vi "USRP_RA_molecularLine_monitor_multSamples.vi"() -> ()   [LabVIEW 2016]
doc: "USRP maser line receiver for amateur radio astronomy."
uses:
  <vilib>/Analysis/4window.llb/windowTd.ctl
  <vilib>/Utility/error.llb/DialogType.ctl
  <vilib>/Analysis/3filter.llb/Filter Passband Type.ctl
  <vilib>/Analysis/2dsp.llb/Power Spectrum (CDB).vi
  <vilib>/Analysis/5stat.llb/RMS (CDB).vi
  <vilib>/Utility/config.llb/Read Key (Double).vi
  <instrlib>/niUSRP/niUSRP Fetch Rx Data (I16).vi
  <vilib>/Analysis/3filter.llb/Butterworth Filter (CDB).vi
  <vilib>/Analysis/0measdsp.llb/Scaled Time Domain Window (CDB).vi
  <vilib>/Utility/file.llb/Write Delimited Spreadsheet (DBL).vi
  <vilib>/Utility/config.llb/Write Key (Double).vi
  <vilib>/Analysis/NI_AALBase.lvlib
  <vilib>/Utility/config.llb/NI_LVConfig.lvlib
  <vilib>/Analysis/NI_AALPro.lvlib
panel:
  in  "Set_mult":bool caption="Set mult"
  in  "Tsys":dbl=150.0 caption="Tsys, K" format="%#_13g"
  in  "Reference Frequency Source":string(combo)="Internal" caption="Ref Freq Source"
  in  "FFT_window":T1=2 caption="FFT window" items=["Rectangle"=0, "Hanning"=1, "Hamming"=2, "Blackman-Harris"=3, "Exact Blackman"=4, "Blackman"=5, "Flat Top"=6, "4 Term B-Harris "=7, "7 Term B-Harris"=8, "Low Sidelobe"=9, "Blackman Nuttall"=11, "Triangle"=30, "Bartlett-Hanning"=31, "Bohman"=32, "Parzen"=33, "Welch"=34, "Kaiser"=60, "Dolph-Chebyshev"=61, "Gaussian"=62]
  out "coerced gain, dB":dbl format="%#_6f"
  in  "Bandwidth_MHz":dbl=2.0 caption="Bandwidth, MHz" min=0.1 max=64.0
  in  "Frequency_MHz":dbl(knob)=1427.4 caption="Frequency, MHz" min=70.0 max=6000.0 scale=70.0..6000.0 scale format="%#1_5g"
  out "Active Antenna":string
  out "Freq (actual)":dbl=1431299999.9970195 format="%#.6p"
  in  "device ID":refnum<k15>="B200miniUSRP"
  out "FFT_error":i32 caption="FFT, proc"
  in  "FFT_size_mult":dbl=50000.0 caption="FFT size av multiplier" min=1.0 max=100000.0 step=1.0 format="%#_8g"
  in  "Power mult":dbl=7e-06 format="%#_13g"
  out "Power_diff":dbl caption="Power diff"
  out "Power_ref":dbl caption="Power ref"
  in  "Power ref":bool
  out "Power_BW":dbl caption="Power in BW"
  out "RMS_error":i32 caption="RMS"
  in  "Pause":bool
  in  "cycle delay, ms":u32
  in  "dB_scale":bool caption="dB scale"
  in  "Reset":bool
  out "TIme elapsed, s":dbl
  in  "Rewrite":bool
  out "Number of av":u32
  in  "File recording":bool
  out "cycle time, s":dbl
  out "Overload":bool
  out "Level":dbl(slide) scale=0.0..1.0 scale format="%#_3g"
  in  "Video_av_on":bool
  in  "Video_av":dbl=500.0 caption="Video Av" min=1.0 max=1000000.0 step=1.0 format="%#_4g"
  in  "DC_block":bool caption="DC block"
  in  "Freq_cutoff_kHz":dbl=10.0 caption="Cutoff, kHz" min=0.01 max=5000.0 step=1.0
  out "RBW":dbl=4.0 caption="RBW, kHz"
  in  "Plot_mult":dbl=0.00020000000000042206 caption="Plot mult" min=0.0 step=5.0
  in  "?":bool
  out "Samplerate":dbl=20000000.0 caption="Sample rate (SR)" min=80000.0 max=40000000.0 step=1.0 format="%#_8g"
  in  "FFT_size":dbl=501.0 caption="FFT size" min=128.0 max=28000000.0 step=1.0 format="%#_8g"
  in  "VGA1_dB":dbl=19.0 caption="Gain, dB" min=-50.0 max=100.0 step=1.0 format="%#_2g"
  out "Spectrum":cluster{dbl, dbl, dbl[]}(graph)={434.616665995587, 1.9999999937668345e-05, array[5000 elements]} caption="Power Spectrum"
  # "errors (0 if OK)"
  # "noise equivalent"
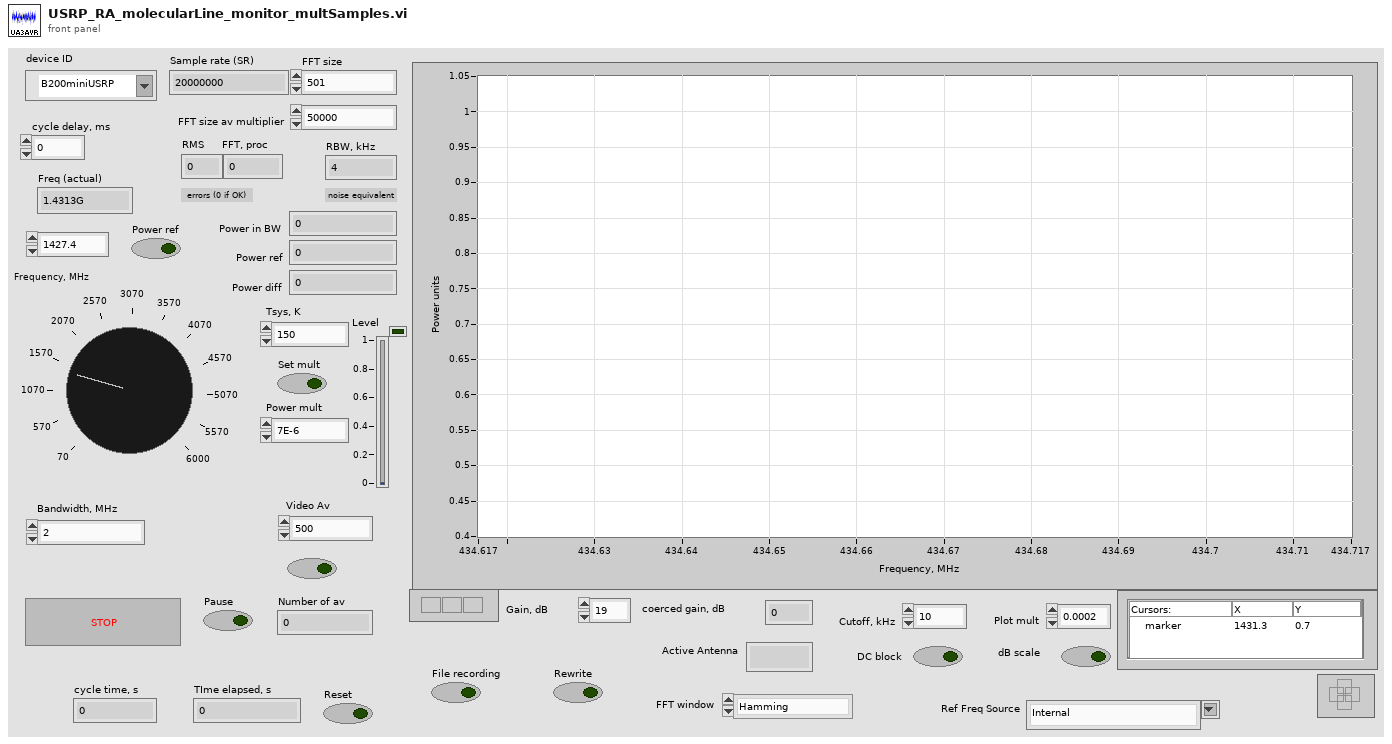
[diagram p1: front panel]
types:
  T1 = typedef "NI_AALPro.lvlib/windowTd.ctl" = u32
  T2 = typedef "DialogType.ctl" = u16
  T3 = typedef "NI_LVConfig.lvlib/Config Data RefNum.ctl" = refnum<k1>
  T4 = typedef "NI_AALBase.lvlib/Filter Passband Type.ctl" = enum32{"Lowpass", "Highpass", "Bandpass", "Bandstop"}
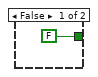
[diagram p3: hidden frame]
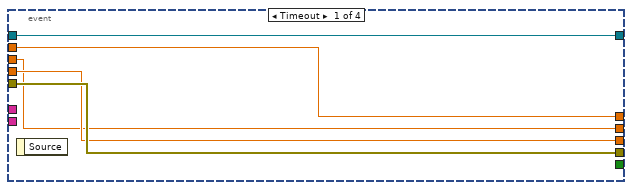
[diagram p4: hidden frame]
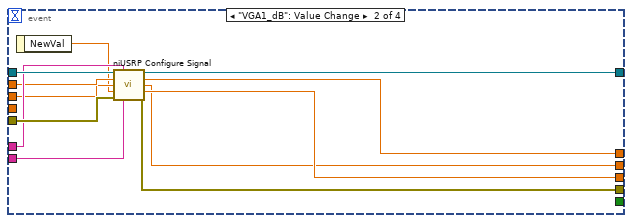
[diagram p5: hidden frame]
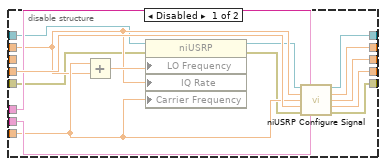
[diagram p6: hidden frame]
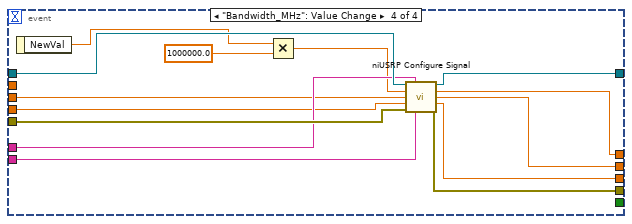
[diagram p7: hidden frame]
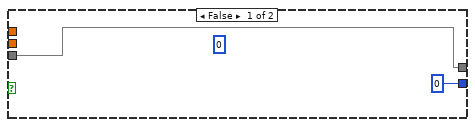
[diagram p8: hidden frame]
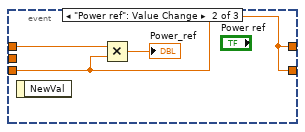
[diagram p9: hidden frame]
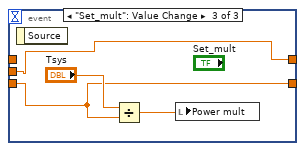
[diagram p10: hidden frame]
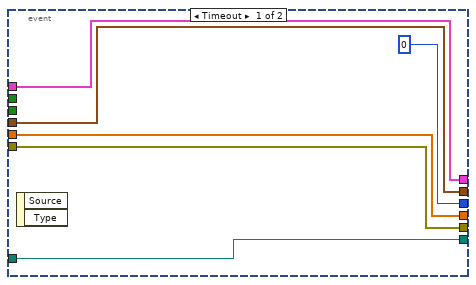
[diagram p11: hidden frame]
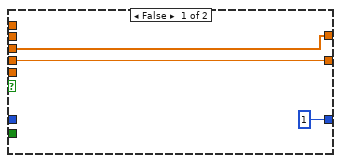
[diagram p13: hidden frame]
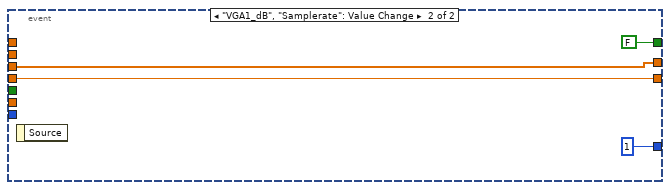
[diagram p15: hidden frame]
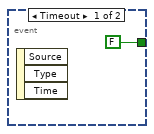
[diagram p16: hidden frame]
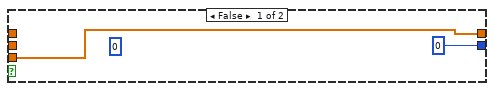
[diagram p17: hidden frame]
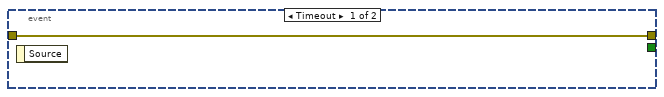
[diagram p18: hidden frame]
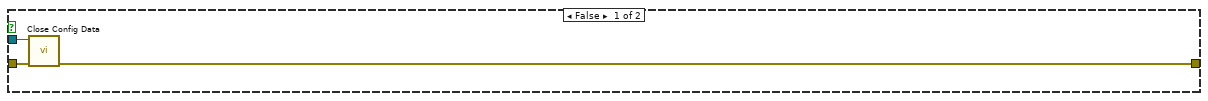
[diagram p20: hidden frame]
diagram:
  w24 = 16 items=["16-bit"=16, "8-bit"=8] ("Sample Width")
  w25 = 1 items=["CDB", "I16"] ("Host Data Type")
  w11 = "0"  # enabled channel
  w45 = T2 3 items=["no dialog", "OK message", "continue or stop message", "OK message + warnings", "continue/stop + warnings"] ("type of dialog (OK msg:1)")
  w53 = TRUE ("use system decimal point (T)")
  w52 = "Data" ("section")
  # "USRP initialization"
  # "Loag CFG values"
  # "Saving file on Stop"
  # "Reading and loading previously saved parameters from CFG-file"
  # "Saving last parameters to CFG-file"
  n1 = call <vilib>:"Application Directory.vi"() -> ("Application Directory"=w78:path)
  n2 = Build Path(base path=w78, name or relative path="USRP_line_monitor.cfg") -> (appended path=w87:path)
  n3 = call <vilib>:"Open Config Data.vi"("create file if necessary (T)"=TRUE, "configuration file path"=w87) -> ("error out"=w84:errorcluster, "file created?"=w82:bool, "refnum"=w86:T3)  [unwired: 7 in]
  n4 = Not(x=w82) -> (.not. x?=w81:bool)
  n5 = case shown="True" w81 {
    tunnel: w86 -> [w95 w131]
    tunnel: w84 -> [w97 w130]
    tunnel: [w96 w129] -> w44
    frame False {
      n6 = call <vilib>:"Close Config Data.vi"("error in (no error)"=w97, "refnum"=w95) -> ("error out"=w96:errorcluster)  [unwired: 8 in, 1 out]
    }
    frame True {
      w108 = "Data" ("section")
      n7 = call-poly <vilib>:"Read Key.vi"("section"=w108, "error in (no error)"=w130, "key"="Frequency_MHz", "refnum"=w131) -> ("error out"=w104:errorcluster, "value"=w102:dbl, "refnum out"=w105:T3)  [unwired: 4 in, 1 out]
      n8 = property on="Frequency_MHz" class="Knob (strict)"(error in=w104, "Value"=w102) -> (error out=w103:errorcluster)  [unwired: 1 in, 1 out]
      n9 = call-poly <vilib>:"Read Key.vi"("section"=w108, "error in (no error)"=w103, "key"="VGA1_dB" ("Control Name"), "refnum"=w105) -> ("error out"=w127:errorcluster, "value"=w128:dbl, "refnum out"=w121:T3)  [unwired: 4 in, 1 out]
      n10 = property on="VGA1_dB" class="DigNum (strict)"(error in=w127, "Value"=w128) -> (error out=w123:errorcluster)  [unwired: 1 in, 1 out]
      n11 = call-poly <vilib>:"Read Key.vi"("section"=w108, "error in (no error)"=w123, "key"="FFT_size" ("Control Name"), "refnum"=w121) -> ("error out"=w125:errorcluster, "value"=w124:dbl, "refnum out"=w119:T3)  [unwired: 4 in, 1 out]
      n12 = property on="FFT_size" class="DigNum (strict)"(error in=w125, "Value"=w124) -> (error out=w120:errorcluster)  [unwired: 1 in, 1 out]
      n13 = call-poly <vilib>:"Read Key.vi"("section"=w108, "error in (no error)"=w120, "key"="Bandwidth_MHz" ("Control Name"), "refnum"=w119) -> ("error out"=w101:errorcluster, "value"=w99:dbl, "refnum out"=w115:T3)  [unwired: 4 in, 1 out]
      n14 = property on="Bandwidth_MHz" class="DigNum (strict)"(error in=w101, "Value"=w99) -> (error out=w100:errorcluster)  [unwired: 1 in, 1 out]
      n15 = call-poly <vilib>:"Read Key.vi"("section"=w108, "error in (no error)"=w100, "key"="Plot_mult" ("Control Name"), "refnum"=w115) -> ("error out"=w117:errorcluster, "value"=w116:dbl, "refnum out"=w109:T3)  [unwired: 4 in, 1 out]
      n16 = property on="Plot_mult" class="DigNum (strict)"(error in=w117, "Value"=w116) -> (error out=w110:errorcluster)  [unwired: 1 in, 1 out]
      n17 = call-poly <vilib>:"Read Key.vi"("section"=w108, "error in (no error)"=w110, "key"="Video_av" ("Control Name"), "refnum"=w109) -> ("error out"=w112:errorcluster, "value"=w111:dbl, "refnum out"=w107:T3)  [unwired: 4 in, 1 out]
      n18 = property on="Video_av" class="DigNum (strict)"(error in=w112, "Value"=w111) -> (error out=w106:errorcluster)  [unwired: 1 in, 1 out]
      n19 = call <vilib>:"Close Config Data.vi"("error in (no error)"=w106, "refnum"=w107) -> ("error out"=w129:errorcluster)  [unwired: 8 in, 1 out]
    }
  }
  n20 = flat-sequence {
    tunnel: w44 -> [w135]
    tunnel: [w135] -> w9
    tunnel: ["VGA1_dB"] -> w8
    tunnel: ["Frequency_MHz"] -> w7
    tunnel: ["Bandwidth_MHz"] -> w6
    frame #0 {
    }
  }
  n21 = Multiply(x=w6, y=1000000.0) -> (x*y=w14:dbl)
  n22 = Multiply(x=w7, y=1000000.0) -> (x*y=w18:dbl)
  n23 = Round To Nearest(number=w14) -> (nearest integer value=w15:dbl)
  n24 = disable-structure shown="Disabled" {
    disable-tunnel: [w138 w139] -> w27
    disable-tunnel: w18 -> [w137 w139]
    disable-tunnel: w15 -> [w136 _]
    frame Disabled {
      n25 = Add(x=w137, y=w136) -> (x+y=w138:dbl)
    }
    frame Enabled {
    }
  }
  n26 = call <instrlib>:"niUSRP Open Rx Session.vi"("device names"="device ID", "reset"=TRUE, "error in (no error)"=w9) -> ("session handle out"=w20:refnum<k15>, "error out"=w30:errorcluster)  [unwired: 11 in]
  n27 = property class="niUSRP"(reference=w20, error in=w30, "Enabled Channels"=w11, "Host Data Type"=w25, "Sample Width"=w24, "Expected Peak"=1.52587890625e-05, "Bandwidth"=60000000.0 ("Configuration:Bandwidth"), "Reference Frequency Source"="Reference Frequency Source", "Timebase Clock Source"="Internal", "Number of Samples Is Finite"=FALSE ("Configuration:Number of Samples Is Finite"), "LO Frequency"=w27, "IQ Rate"=w15, "Carrier Frequency"=w18, "Gain"=w8) -> (reference out=w21:refnum<k15>, error out=w22:errorcluster, "Active Antenna"=w4:string)
  "Active Antenna" <- w4
  n28 = call <vilib>:"Application Directory.vi"() -> ("Application Directory"=w35:path)
  n29 = call <instrlib>:"niUSRP Configure Signal.vi"("session handle"=w21, "channel list"=w11, "IQ rate"=w15, "carrier frequency"=w18, "gain"=w8, "error in (no error)"=w22, "active antenna"=w4) -> ("session handle out"=w12:refnum<k15>, "coerced IQ rate"=w13:dbl, "coerced carrier frequency"=w17:dbl, "coerced gain"=w5:dbl, "error out"=w10:errorcluster)  [unwired: 4 in]
  "Freq (actual)" <- w17
  "coerced gain, dB" <- w5
  n30 = Build Path(base path=w35, name or relative path="samples-data.txt") -> (appended path=w34:path)
  n31 = Get Date/Time In Seconds() -> (seconds since 1Jan1904=w33:timestamp)
  n32 = while {
    tunnel: [w216] -> w2
    shift-right: [w215] -> w74
    shift-left: _ -> [w255]
    tunnel: w34 -> [w220]
    tunnel: w10 -> [w161]
    tunnel: ["File recording"] -> w76
    tunnel: [w217] -> w75
    tunnel: [w214] -> _
    shift-right: [w218] -> _
    shift-left: w33 -> [w225]
    tunnel: [w208] -> w51
    shift-right: [w199] -> _
    shift-left: _ -> [w203]
    shift-right: [w195] -> _
    shift-left: _ -> [w194]
    tunnel: w17 -> [w150]
    tunnel: w13 -> [w153]
    tunnel: w12 -> [w159]
    tunnel: [w174] -> w1
    tunnel: w11 -> [w156]
    tunnel: w5 -> [w147]
    tunnel: w4 -> [w155]
    stop <- w143 stop-if-true
    # "Spectrum processing and indication"
    # "Power in bandwidth indication"
    # "File savings on pause"
    # "Timing"
    # "Noise RBW"
    # "Sampling procedures"
    # "Changing the main parameters on flight"
    # "Power in the bandwidth and overload indication"
    # "Spectrum averaging procedures"
    # "Finish and close BladeRF"
    # "Video averaging"
    n33 = feedback #1(w153) -> (w152:dbl)
    n34 = feedback #2(w150) -> (w149:dbl)
    n35 = feedback #3(w147) -> (w146:dbl)
    n36 = event shown="[2] \"Frequency_MHz\": Value Change" {
      selector: _ -> [_ _ _ _]
      dyn-events: _ -> [_ _ _ _]
      timeout: 0 -> [_ _ _ _]
      tunnel: w161 -> [w270 w282 w286 w330]
      tunnel: [w270 w281 w296 w329] -> w160
      tunnel: w159 -> [w269 w279 w285 w328]
      tunnel: [w269 w280 w295 w327] -> w158
      tunnel: w156 -> [_ w278 w290 w325]
      tunnel: w152 -> [w267 w277 w287 _]
      tunnel: w149 -> [w266 w276 w284 w324]
      tunnel: [w268 w274 w291 w317] -> w148
      tunnel: w146 -> [w268 _ w294 w323]
      tunnel: [w267 w273 w293 w319] -> w154
      tunnel: [w266 w272 w292 w318] -> w151
      tunnel: w155 -> [_ w271 w289 w326]
      tunnel: [_ _ TRUE _] -> w141
      event Timeout {
        n37 = event-data() -> ()  [unwired: 1 in, 1 out]
      }
      event "VGA1_dB": Value Change {
        n38 = event-data() -> ("NewVal"=w275:dbl)  [unwired: 1 in]
        n39 = call <instrlib>:"niUSRP Configure Signal.vi"("session handle"=w279, "channel list"=w278, "IQ rate"=w277, "carrier frequency"=w276, "gain"=w275, "error in (no error)"=w282, "active antenna"=w271) -> ("session handle out"=w280:refnum<k15>, "coerced IQ rate"=w273:dbl, "coerced carrier frequency"=w272:dbl, "coerced gain"=w274:dbl, "error out"=w281:errorcluster)  [unwired: 4 in]
      }
      event "Frequency_MHz": Value Change {
        n40 = event-data() -> ("NewVal"=w288:dbl)  [unwired: 1 in]
        n41 = disable-structure shown="Enabled" {
          disable-tunnel: [w311 w315] -> w296
          disable-tunnel: [w310 w316] -> w295
          disable-tunnel: w294 -> [w309 w312]
          disable-tunnel: [w308 w314] -> w293
          disable-tunnel: [w307 w313] -> w292
          disable-tunnel: [w306 w312] -> w291
          disable-tunnel: w290 -> [w305 _]
          disable-tunnel: w289 -> [w304 _]
          disable-tunnel: w288 -> [w302 _]
          disable-tunnel: w287 -> [w301 w314]
          disable-tunnel: w286 -> [w300 w315]
          disable-tunnel: w285 -> [w298 w316]
          disable-tunnel: w284 -> [_ w313]
          frame Disabled {
            n42 = Add(x=w302, y=w301) -> (x+y=w303:dbl)
            n43 = property class="niUSRP"(reference=w298, error in=w300, "LO Frequency"=w303, "IQ Rate"=w301, "Carrier Frequency"=w302) -> (reference out=w297:refnum<k15>, error out=w299:errorcluster)
            n44 = call <instrlib>:"niUSRP Configure Signal.vi"("session handle"=w297, "channel list"=w305, "IQ rate"=w301, "carrier frequency"=w302, "gain"=w309, "error in (no error)"=w299, "active antenna"=w304) -> ("session handle out"=w310:refnum<k15>, "coerced IQ rate"=w308:dbl, "coerced carrier frequency"=w307:dbl, "coerced gain"=w306:dbl, "error out"=w311:errorcluster)  [unwired: 4 in]
          }
          frame Enabled {
          }
        }
      }
      event "Bandwidth_MHz": Value Change {
        n45 = event-data() -> ("NewVal"=w322:dbl)  [unwired: 1 in]
        n46 = Multiply(x=w322, y=1000000.0) -> (x*y=w320:dbl)
        n47 = call <instrlib>:"niUSRP Configure Signal.vi"("session handle"=w328, "channel list"=w325, "IQ rate"=w320, "carrier frequency"=w324, "gain"=w323, "error in (no error)"=w330, "active antenna"=w326) -> ("session handle out"=w327:refnum<k15>, "coerced IQ rate"=w319:dbl, "coerced carrier frequency"=w318:dbl, "coerced gain"=w317:dbl, "error out"=w329:errorcluster)  [unwired: 4 in]
      }
    }
    n48 = feedback-in #1(w154) -> ()
    n49 = feedback-in #2(w151) -> ()
    n50 = feedback-in #3(w148) -> ()
    n51 = Round To Nearest(number="FFT_size") -> (nearest integer value=w193:dbl)
    n52 = Divide(x=w152, y=w193) -> (x/y=w260:dbl)
    n53 = Multiply(x="FFT_size_mult", y=w193) -> (x*y=w192:dbl)
    n54 = To Long Integer(number="FFT_size_mult") -> (32bit integer=w191:i32)
    n55 = To Quad Integer(1:w192) -> (0:w168:i64)
    n56 = case shown="True" w141 {
      tunnel: [FALSE ("T button?") w264] -> w140
      frame False {
      }
      frame True {
        n57 = Two Button Dialog(message="The application will be stopped. To change a frequency, please, start it again.") -> (T button?=w264:bool)  [unwired: 2 in]
      }
    }
    n58 = local write "Freq (actual)"(w151) -> ()
    n59 = local write "Samplerate"(w154) -> ()
    n60 = local write "coerced gain, dB"(w148) -> ()
    n61 = call <instrlib>:"niUSRP Configure Number of Samples.vi"("session handle"=w158, "number of samples is finite"=TRUE, "number of samples"=w168, "error in (no error)"=w160) -> ("session handle out"=w165:refnum<k15>, "error out"=w167:errorcluster)  [unwired: 10 in]
    n62 = call <instrlib>:"niUSRP Initiate.vi"("session handle"=w165, "error in (no error)"=w167) -> ("session handle out"=w164:refnum<k15>, "error out"=w166:errorcluster)  [unwired: 12 in]
    n63 = event shown="[1] \"FFT_size\": Value Change" {
      selector: _ -> [_ _]
      dyn-events: _ -> [_ _]
      timeout: 0 -> [_ _]
      tunnel: [FALSE TRUE] -> w178
      event Timeout {
        n64 = event-data() -> ()  [unwired: 1 in, 3 out]
      }
      event "FFT_size": Value Change {
        n65 = event-data() -> ()  [unwired: 1 in, 3 out]
      }
    }
    n66 = call-poly <instrlib>:"niUSRP Fetch Rx Data (poly).vi"("session handle"=w164, "channel list"=w156, "number of samples"=w168, "error in (no error)"=w166) -> ("session handle out"=w176:refnum<k15>, "data"=w173:i16[], "error out"=w177:errorcluster)  [unwired: 8 in, 1 out]
    n67 = To Long Integer(number=w193) -> (32bit integer=w190:i32)
    n68 = Decimate 1D Array(w173) -> (w172:i16[], w171:i16[])
    n69 = call <instrlib>:"niUSRP Abort.vi"("session handle"=w176, "error in (no error)"=w177) -> ("session handle out"=w174:refnum<k15>, "error out"=w175:errorcluster)  [unwired: 12 in]
    n70 = Re/Im To Complex(1:w171, 2:w172) -> (0:w170:cdb[])
    n71 = Initialize Array(0.0 ("element"), w190) -> (w182:dbl[])
    n72 = for {
      N: w191 -> [_]
      tunnel: w170 -> [w352]
      tunnel: w190 -> [w350]
      shift-right: [w331] -> w179
      shift-left: w182 -> [w337]
      tunnel: w152 -> [w348]
      shift-right: [w343] -> w188
      shift-left: _ -> [_]
      shift-right: [w341] -> w187
      shift-left: _ -> [_]
      shift-right: [w342] -> w186
      shift-left: _ -> [_]
      shift-right: [w340] -> w185
      shift-left: _ -> [_]
      tunnel: "DC_block" -> [w339]
      tunnel: "Freq_cutoff_kHz" -> [w338]
      i -> [w336]
      # "Averaging"
      # "Array division"
      # "Windowing and FFT"
      n73 = Multiply(x=w350, y=w336) -> (x*y=w351:i32)
      n74 = To Double Precision Float(number=w336) -> (double precision float=w333:dbl)
      n75 = Multiply(x=w337, y=w333) -> (x*y=w335:dbl[])
      n76 = Array Subset(array=w352, index=w351, length=w350) -> (w349:cdb[])
      n77 = case shown="True" w339 {
        tunnel: w349 -> [w354 w362]
        tunnel: w348 -> [_ w361]
        tunnel: [0 ("error") w360] -> w343
        tunnel: [w354 w359] -> w346
        tunnel: w338 -> [_ w355]
        frame False {
          (unwired) 0 ("error")
        }
        frame True {
          # "DC block"
          n78 = Multiply(x=1000.0, y=w355) -> (x*y=w357:dbl)
          n79 = call-poly <vilib>:"Butterworth Filter.vi"("filter type"=Filter_Passband_Type."Highpass", "low cutoff freq: fl"=w357, "sampling freq: fs"=w361, "X"=w362) -> ("error"=w360:i32, "Filtered X"=w359:cdb[])  [unwired: 4 in]
        }
      }
      n80 = Increment(x=w333) -> (x+1=w332:dbl)
      n81 = call-poly <vilib>:"Scaled Time Domain Window.vi"("window"="FFT_window", "X"=w346) -> ("error"=w341:i32, "window properties"=w340:cluster{"eq noise BW":dbl, "coherent gain":dbl}, "Windowed X"=w345:cdb[])  [unwired: 7 in]
      n82 = call-poly <vilib>:"Power Spectrum.vi"("X"=w345) -> ("Power Spectrum"=w344:dbl[], "error"=w342:i32)
      n83 = Add(x=w335, y=w344) -> (x+y=w334:dbl[])
      n84 = Divide(x=w334, y=w332) -> (x/y=w331:dbl[])
    }
    n85 = case shown="True" "DC_block" {
      tunnel: w170 -> [w456 w464]
      tunnel: w152 -> [_ w463]
      tunnel: [0 ("error") w462] -> w181
      tunnel: [w456 w461] -> w202
      tunnel: "Freq_cutoff_kHz" -> [_ w457]
      frame False {
        (unwired) 0 ("error")
      }
      frame True {
        # "DC block"
        n86 = Multiply(x=1000.0, y=w457) -> (x*y=w459:dbl)
        n87 = call-poly <vilib>:"Butterworth Filter.vi"("filter type"=Filter_Passband_Type."Highpass", "low cutoff freq: fl"=w459, "sampling freq: fs"=w463, "X"=w464) -> ("error"=w462:i32, "Filtered X"=w461:cdb[])  [unwired: 4 in]
      }
    }
    n88 = event shown="[1] Panel Close?" {
      selector: _ -> [_ _]
      dyn-events: _ -> [_ _]
      timeout: 0 -> [_ _]
      tunnel: [_ w467] -> w144
      tunnel: [w465 w466] -> w145
      tunnel: w175 -> [w465 w466]
      event Timeout {
        n89 = event-data() -> ()  [unwired: 1 in, 1 out]
      }
      event Panel Close? {
        n90 = event-data() -> ()  [unwired: 1 in, 1 out]
        n91 = Two Button Dialog(message="Stop BladeRF & close window?") -> (T button?=w467:bool)  [unwired: 2 in]
        n92 = Not(x=w467) -> (.not. x?=w468:bool)
        n93 = event-data("Discard?"=w468) -> ()  [unwired: 1 in, 1 out]
      }
    }
    n94 = Select(t=w182, s=w178, f=w255) -> (s? t:f=w257:dbl[])
    n95 = Decimate 1D Array(w202) -> (w201:cdb[])  [unwired: 1 out]
    n96 = Complex To Re/Im(x + iy=w202) -> (x=w241:dbl[], y=w240:dbl[])
    n97 = Absolute Value(x=w241) -> (abs(x)=w242:dbl[])
    n98 = Absolute Value(x=w240) -> (abs(x)=w239:dbl[])
    n99 = call-poly <vilib>:"RMS.vi"("X"=w201) -> ("rms value"=w207:dbl, "error"=→"RMS_error":i32)
    n100 = Array Max & Min(array=w242) -> (max value=w244:dbl)  [unwired: 3 out]
    n101 = Array Max & Min(array=w239) -> (max value=w245:dbl)  [unwired: 3 out]
    n102 = Compound Arithmetic op=OR(w145, w144, "?") -> (w142:bool)
    n103 = Greater Or Equal?(x=w244, y=w245) -> (x >= y?=w246:bool)
    n104 = Or(x=w142, y=w140) -> (x .or. y?=w143:bool)
    n105 = Select(t=w244, s=w246, f=w245) -> (s? t:f=w243:dbl)
    n106 = Scale By Power Of 2(n=i16 -15, x=w243) -> (x*2^n=w163:dbl)
    "Level" <- w163
    n107 = Greater?(x=w163, y=0.9) -> (0:→"Overload":bool)
    n108 = Square(x=w207) -> (x^2=w205:dbl)
    n109 = Unbundle By Name(w185) -> ("eq noise BW"=w232:dbl)
    n110 = Compound Arithmetic op=ADD(w181, w188, w187, w186) -> (→"FFT_error":i32)
    n111 = Multiply(x=w232, y=0.001) -> (x*y=w233:dbl)
    n112 = Multiply(x=w260, y=w233) -> (x*y=→"RBW":dbl)
    n113 = feedback #4(TRUE) -> (w247:bool)
    n114 = And(x="Video_av_on", y=w247) -> (x .and. y?=w249:bool)
    n115 = feedback #5(u32 1) -> (w227:u32)
    n116 = event shown="[0] Timeout" {
      selector: _ -> [_ _]
      dyn-events: _ -> [_ _]
      timeout: 0 -> [_ _]
      tunnel: w179 -> [w426 w451]
      tunnel: w257 -> [w425 _]
      tunnel: "Video_av" -> [w417 _]
      tunnel: w249 -> [w424 _]
      tunnel: [w423 w451] -> w237
      tunnel: [TRUE FALSE] -> w248
      tunnel: w227 -> [w418 _]
      tunnel: [w421 u32 1] -> w230
      tunnel: w205 -> [w414 w449]
      tunnel: w203 -> [w413 _]
      tunnel: [w412 w449] -> w200
      event Timeout {
        n117 = event-data() -> ()  [unwired: 1 in, 1 out]
        n118 = To Double Precision Float(number=w418) -> (double precision float=w416:dbl)
        n119 = Not Equal?(x=w417, y=w416) -> (x != y?=w415:bool)
        n120 = In Range and Coerce(upper limit=w417, x=w416, lower limit=1.0) -> (coerced(x)=w420:dbl)  [unwired: 1 out]
        n121 = case shown="True" w424 {
          tunnel: w426 -> [w429 w440]
          tunnel: [w429 w443] -> w423
          tunnel: w425 -> [_ w442]
          tunnel: w420 -> [_ w434]
          tunnel: w418 -> [_ w439]
          tunnel: [u32 1 w438] -> w421
          tunnel: w415 -> [_ w437]
          tunnel: w414 -> [w427 w432]
          tunnel: w413 -> [_ w431]
          tunnel: [w427 w430] -> w412
          frame False {
          }
          frame True {
            n122 = case shown="True" w437 {
              tunnel: w439 -> [w446 w448]
              tunnel: [w446 w447] -> w438
              frame False {
              }
              frame True {
                n123 = Increment(x=w448) -> (x+1=w447:u32)
              }
            }
            n124 = Subtract(x=w434, y=1.0) -> (x-y=w433:dbl)
            n125 = Multiply(x=w431, y=w433) -> (x*y=w436:dbl)
            n126 = Multiply(x=w442, y=w433) -> (x*y=w445:dbl[])
            n127 = Add(x=w440, y=w445) -> (x+y=w444:dbl[])
            n128 = Add(x=w432, y=w436) -> (x+y=w435:dbl)
            n129 = Divide(x=w444, y=w434) -> (x/y=w443:dbl[])
            n130 = Divide(x=w435, y=w434) -> (x/y=w430:dbl)
          }
        }
      }
      event "VGA1_dB", "Samplerate": Value Change {
        n131 = event-data() -> ()  [unwired: 1 in, 1 out]
      }
    }
    "Number of av" <- w230
    n132 = feedback-in #4(w248) -> ()
    n133 = feedback-in #5(w230) -> ()
    n134 = Multiply(x="Power mult", y=w200) -> (x*y=→"Power_BW":dbl)
    n135 = flat-sequence {
      tunnel: w145 -> [w410]
      tunnel: w237 -> [w411]
      tunnel: [w411] -> w222
      tunnel: [w410] -> w221
      tunnel: [w409] -> w235
      tunnel: [w406] -> w226
      tunnel: w225 -> [w403]
      tunnel: [w402] -> w219
      frame #0 {
        n136 = Get Date/Time In Seconds() -> (seconds since 1Jan1904=w404:timestamp)
        n137 = Select(t=w404, s="Reset", f=w403) -> (s? t:f=w402:timestamp)
        n138 = Wait (ms)(milliseconds to wait="cycle delay, ms") -> ()  [unwired: 1 out]
        n139 = To Double Precision Float(number=w404) -> (double precision float=w407:dbl)
        n140 = To Double Precision Float(number=w402) -> (double precision float=w408:dbl)
        n141 = Subtract(x=w407, y=w408) -> (x-y=w406:dbl)
        n142 = call <vilib>:"High Resolution Relative Seconds.vi"() -> ("relative seconds"=w409:dbl)
      }
    }
    n143 = event shown="[0] Timeout" {
      selector: _ -> [_ _ _]
      dyn-events: _ -> [_ _ _]
      timeout: 0 -> [_ _ _]
      tunnel: w200 -> [w366 w368 w372]
      tunnel: [w366 w368 w372] -> w199
      tunnel: "Power mult" -> [w364 w369 _]
      tunnel: [w363 w368 w371] -> w195
      tunnel: w194 -> [w363 _ w371]
      event Timeout {
        n144 = event-data() -> ()  [unwired: 1 in, 1 out]
        n145 = Subtract(x=w366, y=w363) -> (x-y=w367:dbl)
        n146 = Multiply(x=w364, y=w367) -> (x*y=→"Power_diff":dbl)
      }
      event "Power ref": Value Change {
        n147 = event-data() -> ()  [unwired: 1 in, 1 out]
        n148 = Multiply(x=w369, y=w368) -> (x*y=→"Power_ref":dbl)
      }
      event "Set_mult": Value Change {
        n149 = event-data() -> ()  [unwired: 1 in, 1 out]
        n150 = Divide(x="Tsys", y=w372) -> (x/y=w374:dbl)
        n151 = local write "Power mult"(w374) -> ()
      }
    }
    n152 = call "Spectrum_data_bundle_Jy_linear.vi"("FFT size"=w193, "Power spectrum input"=w237, "dB_scale"="dB_scale", "Central frequency, Hz"=w149, "Sample Rate"=w152, "Plot mult"="Plot_mult") -> ("Output cluster to waveform graph"=w223:cluster{dbl, dbl, dbl[]})  [unwired: 5 in]
    "Spectrum" <- w223
    n153 = Not(x="Rewrite") -> (.not. x?=w208:bool)
    n154 = feedback-in #6(w235) -> ()
    n155 = feedback #6() -> (w234:dbl)  [unwired: 1 in]
    n156 = Subtract(x=w235, y=w234) -> (x-y=→"cycle time, s":dbl)
    n157 = feedback #7(0 ("t")) -> (w211:i32)
    n158 = event shown="[1] \"Pause\": Value Change" {
      selector: _ -> [_ _]
      dyn-events: _ -> [_ _]
      timeout: w211 -> [_ _]
      tunnel: w223 -> [w380 w389]
      tunnel: [w380 w389] -> w214
      tunnel: w222 -> [w377 w390]
      tunnel: [w377 w390] -> w215
      tunnel: w221 -> [w376 w392]
      tunnel: [w376 w391] -> w216
      tunnel: w220 -> [w379 w393]
      tunnel: [w379 w393] -> w217
      tunnel: w219 -> [w378 w388]
      tunnel: [w378 w388] -> w218
      tunnel: "File recording" -> [_ w382]
      tunnel: [0 ("t") w384] -> w212
      tunnel: w208 -> [_ w381]
      event Timeout {
        n159 = event-data() -> ()  [unwired: 1 in, 2 out]
      }
      event "Pause": Value Change {
        n160 = event-data() -> ("NewVal"=w387:bool)  [unwired: 1 in, 1 out]
        n161 = And(x=w382, y=w387) -> (x .and. y?=w383:bool)
        n162 = Select(t=-1, s=w387, f=0) -> (s? t:f=w384:i32)
        n163 = case shown="True" w383 {
          tunnel: [w394 w400] -> w391
          tunnel: w392 -> [w394 w399]
          tunnel: w390 -> [_ w396]
          tunnel: w381 -> [_ w395]
          frame False {
          }
          frame True {
            n164 = call-poly <vilib>:"Write Delimited Spreadsheet.vi"("format (%.3f)"="%.5e", "1D data"=w396, "append to file? (new file:F)"=w395, "error in (no error)"=w399, "delimiter (\\t)"="," ("delimiter (\\t)")) -> ("error out"=w400:errorcluster)  [unwired: 9 in, 1 out]
          }
        }
      }
    }
    n165 = feedback-in #7(w212) -> ()
    "Samplerate" <- w153
    "TIme elapsed, s" <- w226
  }
  n166 = call <instrlib>:"niUSRP Close Session.vi"("session handle"=w1, "error in (no error)"=w2) -> ("error out"=w77:errorcluster)  [unwired: 13 in]
  n167 = case shown="True" w76 {
    tunnel: [w470 w476] -> w37
    tunnel: w75 -> [_ _]
    tunnel: w77 -> [w470 w475]
    tunnel: w74 -> [_ w472]
    tunnel: w51 -> [_ w471]
    frame False {
    }
    frame True {
      n168 = call-poly <vilib>:"Write Delimited Spreadsheet.vi"("format (%.3f)"="%.5e", "1D data"=w472, "append to file? (new file:F)"=w471, "error in (no error)"=w475, "delimiter (\\t)"="," ("delimiter (\\t)")) -> ("error out"=w476:errorcluster)  [unwired: 9 in, 1 out]
    }
  }
  n169 = call <vilib>:"Simple Error Handler.vi"("type of dialog (OK msg:1)"=w45, "error in (no error)"=w37) -> ("error out"=w80:errorcluster)  [unwired: 3 in, 4 out]
  n170 = call <vilib>:"Application Directory.vi"() -> ("Application Directory"=w85:path)
  n171 = call <vilib>:"Clear Errors.vi"("error in (no error)"=w80) -> ("error out"=w79:errorcluster)  [unwired: 5 in, 1 out]
  n172 = Build Path(base path=w85, name or relative path="USRP_line_monitor.cfg") -> (appended path=w89:path)
  n173 = call <vilib>:"Open Config Data.vi"("error in (no error)"=w79, "create file if necessary (T)"=TRUE, "configuration file path"=w89) -> ("error out"=w46:errorcluster, "refnum"=w94:T3)  [unwired: 6 in, 1 out]
  n174 = property on="Frequency_MHz" class="Knob (strict)"(error in=w46) -> (error out=w40:errorcluster, "Value"=w39:dbl)  [unwired: 1 in, 1 out]
  n175 = call-poly <vilib>:"Write Key.vi"("use system decimal point (T)"=w53, "section"=w52, "error in (no error)"=w40, "value"=w39, "key"="Frequency_MHz", "refnum"=w94) -> ("error out"=w49:errorcluster, "refnum out"=w50:T3)  [unwired: 3 in, 1 out]
  n176 = property on="VGA1_dB" class="DigNum (strict)"(error in=w49) -> (error out=w71:errorcluster, "Value"=w72:dbl)  [unwired: 1 in, 1 out]
  n177 = call-poly <vilib>:"Write Key.vi"("use system decimal point (T)"=w53, "section"=w52, "error in (no error)"=w71, "value"=w72, "key"="VGA1_dB" ("Control Name"), "refnum"=w50) -> ("error out"=w63:errorcluster, "refnum out"=w61:T3)  [unwired: 3 in, 1 out]
  n178 = property on="FFT_size" class="DigNum (strict)"(error in=w63) -> (error out=w66:errorcluster, "Value"=w67:dbl)  [unwired: 1 in, 1 out]
  n179 = call-poly <vilib>:"Write Key.vi"("use system decimal point (T)"=w53, "section"=w52, "error in (no error)"=w66, "value"=w67, "key"="FFT_size" ("Control Name"), "refnum"=w61) -> ("error out"=w43:errorcluster, "refnum out"=w60:T3)  [unwired: 3 in, 1 out]
  n180 = property on="Bandwidth_MHz" class="DigNum (strict)"(error in=w43) -> (error out=w42:errorcluster, "Value"=w41:dbl)  [unwired: 1 in, 1 out]
  n181 = call-poly <vilib>:"Write Key.vi"("use system decimal point (T)"=w53, "section"=w52, "error in (no error)"=w42, "value"=w41, "key"="Bandwidth_MHz" ("Control Name"), "refnum"=w60) -> ("error out"=w62:errorcluster, "refnum out"=w59:T3)  [unwired: 3 in, 1 out]
  n182 = property on="Plot_mult" class="DigNum (strict)"(error in=w62) -> (error out=w68:errorcluster, "Value"=w69:dbl)  [unwired: 1 in, 1 out]
  n183 = call-poly <vilib>:"Write Key.vi"("use system decimal point (T)"=w53, "section"=w52, "error in (no error)"=w68, "value"=w69, "key"="Plot_mult" ("Control Name"), "refnum"=w59) -> ("error out"=w55:errorcluster, "refnum out"=w54:T3)  [unwired: 3 in, 1 out]
  n184 = property on="Video_av" class="DigNum (strict)"(error in=w55) -> (error out=w56:errorcluster, "Value"=w57:dbl)  [unwired: 1 in, 1 out]
  n185 = call-poly <vilib>:"Write Key.vi"("use system decimal point (T)"=w53, "section"=w52, "error in (no error)"=w56, "value"=w57, "key"="Video_av" ("Control Name"), "refnum"=w54) -> ("error out"=w48:errorcluster, "refnum out"=w47:T3)  [unwired: 3 in, 1 out]
  n186 = call <vilib>:"Close Config Data.vi"("error in (no error)"=w48, "write file if changed (T)"=TRUE, "refnum"=w47) -> ("error out"=w93:errorcluster)  [unwired: 7 in, 1 out]
  n187 = call <vilib>:"Simple Error Handler.vi"("error in (no error)"=w93) -> ()  [unwired: 4 in, 5 out]
